vi "magic.vi"(8 "error in":errorcluster, 11 "payload":string) -> (0 "error out":errorcluster, 3 "body":string)   [LabVIEW 2020]
uses:
  <vilib>/httpClient/POSTBuffer.vi
  <vilib>/httpClient/PUTBuffer.vi
  <vilib>/httpClient/LabVIEWHTTPClient.lvlib
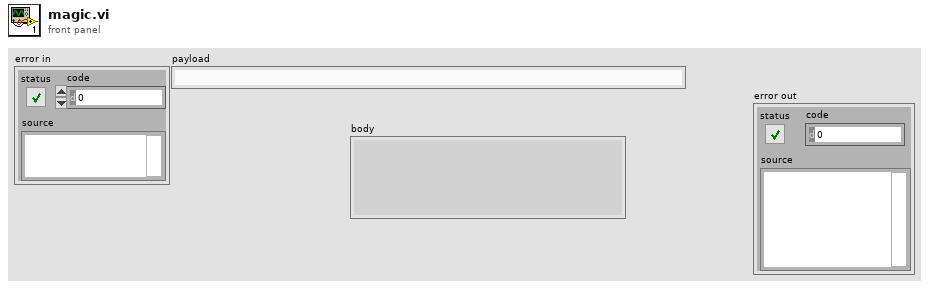
[diagram p1: front panel]
types:
  T1 = typedef "LabVIEWHTTPClient.lvlib/ClientHandle.ctl" = refnum<k1>
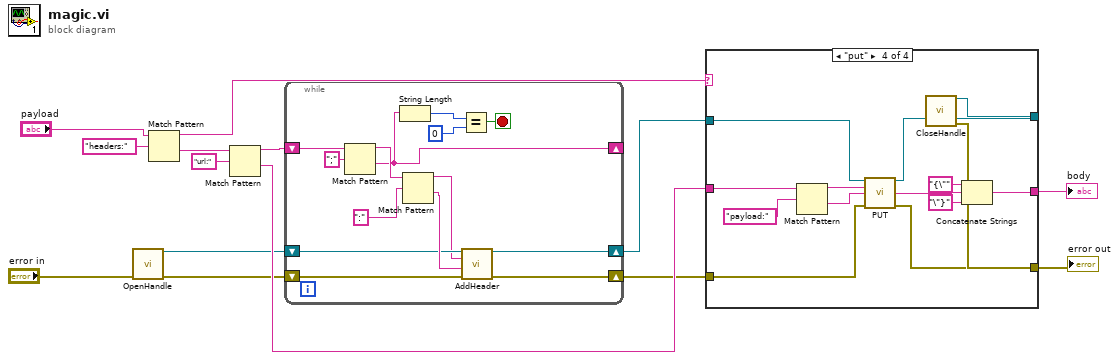
[diagram p0: block diagram]
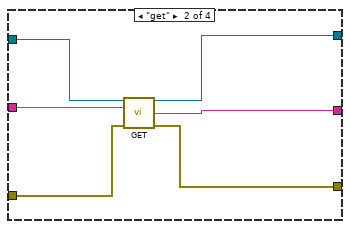
[diagram p3: hidden frame]
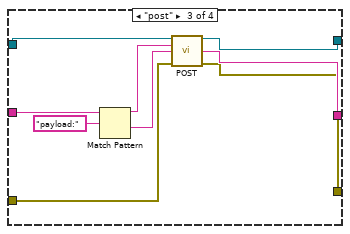
[diagram p4: hidden frame]
diagram:
  n1 = call <vilib>:"OpenHandle.vi"("error in (no error)"="error in") -> ("client handle out"=w4:T1, "error out"=w2:errorcluster)  [unwired: 13 in]
  n2 = Match Pattern(string="payload", regular expression="headers:") -> (before substring=w8:string, after substring=w9:string)  [unwired: 1 in, 2 out]
  n3 = Match Pattern(string=w9, regular expression="url:") -> (before substring=w5:string, after substring=w6:string)  [unwired: 1 in, 2 out]
  n4 = while {
    shift-right: [w19] -> _
    shift-left: w5 -> [w28]
    shift-right: [w23] -> w3
    shift-left: w4 -> [w24]
    shift-right: [w21] -> w1
    shift-left: w2 -> [w22]
    stop <- w16 stop-if-true
    n5 = Match Pattern(string=w28, regular expression=";") -> (before substring=w27:string, after substring=w19:string)  [unwired: 1 in, 2 out]
    n6 = String Length(string=w19) -> (length=w18:i32)
    n7 = Match Pattern(string=w27, regular expression=":") -> (before substring=w20:string, after substring=w25:string)  [unwired: 1 in, 2 out]
    n8 = Equal?(x=w18, y=0) -> (x = y?=w16:bool)
    n9 = call <vilib>:"AddHeader.vi"("client handle"=w24, "header"=w20, "value"=w25, "error in (no error)"=w22) -> ("client handle out"=w23:T1, "error out"=w21:errorcluster)  [unwired: 10 in]
  }
  n10 = case shown="\"put\"" w8 {
    tunnel: [w30 w37 w46 w58] -> w7
    tunnel: w6 -> [_ w36 w40 w53]
    tunnel: [_ w35 w45 w50] -> w13
    tunnel: w1 -> [w31 w34 w44 w57]
    tunnel: [w31 w33 w43 w56] -> w12
    tunnel: w3 -> [w30 w32 w42 w55]
    frame Default {
    }
    frame "get" {
      n11 = call <vilib>:"GET.vi"("client handle"=w32, "url"=w36, "error in (no error)"=w34) -> ("client handle out"=w37:T1, "body"=w35:string, "error out"=w33:errorcluster)  [unwired: 9 in, 1 out]
    }
    frame "post" {
      n12 = Match Pattern(string=w40, regular expression="payload:") -> (before substring=w39:string, after substring=w38:string)  [unwired: 1 in, 2 out]
      n13 = call-poly <vilib>:"POST.vi"("client handle"=w42, "url"=w39, "buffer"=w38, "error in (no error)"=w44) -> ("client handle out"=w46:T1, "body"=w45:string, "error out"=w43:errorcluster)  [unwired: 8 in, 1 out]
    }
    frame "put" {
      n14 = Match Pattern(string=w53, regular expression="payload:") -> (before substring=w52:string, after substring=w51:string)  [unwired: 1 in, 2 out]
      n15 = call-poly <vilib>:"PUT.vi"("client handle"=w55, "url"=w52, "buffer"=w51, "error in (no error)"=w57) -> ("client handle out"=w58:T1, "body"=w49:string, "error out"=w56:errorcluster)  [unwired: 8 in, 1 out]
      n16 = Concatenate Strings("{\"" ("string"), w49, "\"}" ("string")) -> (w50:string)
    }
  }
  "body" <- w13
  "error out" <- w12
  n17 = call <vilib>:"CloseHandle.vi"("client handle"=w7, "error in (no error)"=w12) -> ()  [unwired: 13 in, 1 out]
